vi "Write File.vi"(8 "error in":errorcluster, 10 "Data In":refnum<class "Data.lvclass">, 11 "File Obs in":refnum<class "CRD File Obs.lvclass">) -> (0 "error out":errorcluster, 3 "File Obs out":refnum<class "CRD File Obs.lvclass">)   [LabVIEW 2014, in "CRD File Obs.lvclass"]
uses:
  CRD File Obs.lvclass
  Data/Main/crd_data_enum.ctl
  Data/Main/CRDS Data.lvclass
  Data/Data.lvclass
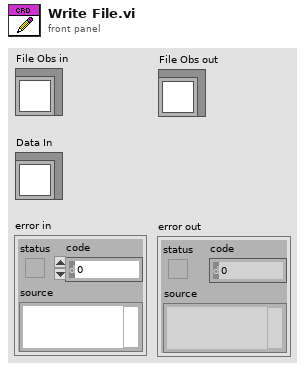
[diagram p1: front panel]
types:
  T1 = typedef "crd_data_enum.ctl" = enum8{"Time", "RHw", "TRH", "P", "Tmean", "RHsense", "TQ", "PQ", "Q", "Q0", "Qcal", "Qset", "extDilFac", "taucorr", "tau0corr", "stdevtau", "ext", "extCorr", "etau", "tau", "tau0", "Purge_Data", "NoData", "reserved", "Ttec", "Ang Exp", "Gamma", "filter", "fOverride", "notes", "max amp", "Tthermistor", "RhdilFac", "Psense", "TRHsense_bank", "RHsense_bank", "MFC_Data", "Thum", "ThumSP", "O3 Flow", "Pinlet Flow", "CLAP Flow", "O3 Add Valve", "O2 Valve", "O3 Cal"}
  T2 = enum16{"big-endian, network order", "native, host order", "little-endian"}
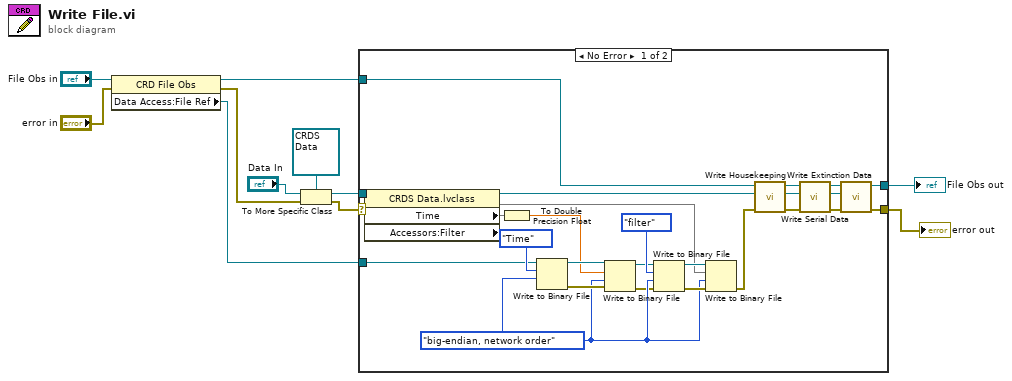
[diagram p0: block diagram]
diagram:
  n1 = property class="CRD File Obs"(reference="File Obs in", error in="error in") -> (reference out=w6:refnum<class "CRD File Obs.lvclass">, error out=w3:errorcluster, "Data Access:File Ref"=w7:refnum<file>)
  n2 = To More Specific Class(target class=refnum<class "CRDS Data.lvclass"> refnum ("CRDS Data in"), reference="Data In", error in=w3) -> (specific class reference=w9:refnum<class "CRDS Data.lvclass">, error out=w2:errorcluster)
  n3 = case shown="No Error" w2 {
    selector: w2 -> [w14 w39]
    tunnel: [w16 w39] -> w4
    tunnel: w9 -> [w30 _]
    tunnel: w7 -> [w13 _]
    tunnel: w6 -> [w24 w38]
    tunnel: [w15 w38] -> w5
    frame No Error {
      w28 = T2."big-endian, network order" ("byte order (0:big-endian, network order)")
      n4 = property class="CRDS Data.lvclass"(reference=w30, error in=w14) -> (reference out=w25:refnum<class "CRDS Data.lvclass">, "Time"=w29, "Accessors:Filter"=w12)  [unwired: 1 out]
      n5 = To Double Precision Float(number=w29) -> (double precision float=w34:dbl)
      n6 = Write to Binary File(file (use dialog)=w13, data=crd_data_enum."Time" ("CRD_Data_Enum"), 9:w28) -> (refnum out=w35:refnum<file>, error out=w36:errorcluster)  [unwired: 3 in, 1 out]
      n7 = Write to Binary File(file (use dialog)=w35, data=w34, error in=w36, 9:w28) -> (refnum out=w27:refnum<file>, error out=w26:errorcluster)  [unwired: 2 in, 1 out]
      n8 = Write to Binary File(file (use dialog)=w27, data=crd_data_enum."filter" ("CRD_Data_Enum"), error in=w26, 9:w28) -> (refnum out=w32:refnum<file>, error out=w31:errorcluster)  [unwired: 2 in, 1 out]
      n9 = Write to Binary File(file (use dialog)=w32, data=w12, error in=w31, 9:w28) -> (error out=w20:errorcluster)  [unwired: 2 in, 2 out]
      n10 = call "Write Housekeeping.vi"("error in"=w20, "CRDS Data in"=w25, "File Obs in"=w24) -> ("error out"=w21:errorcluster, "CRD Data Out"=w23:refnum<class "CRDS Data.lvclass">, "File Obs Out"=w22:refnum<class "CRD File Obs.lvclass">)  [unwired: 6 in]
      n11 = call "Write Serial Data.vi"("error in"=w21, "CRD Data In"=w23, "File Obs in"=w22) -> ("error out"=w17:errorcluster, "CRD Data Out"=w18:refnum<class "CRDS Data.lvclass">, "File Obs Out"=w19:refnum<class "CRD File Obs.lvclass">)  [unwired: 6 in]
      n12 = call "Write Extinction Data.vi"("error in"=w17, "CRDS Data in"=w18, "CRD File Obs in"=w19) -> ("error out"=w16:errorcluster, "CRD File Obs out"=w15:refnum<class "CRD File Obs.lvclass">)  [unwired: 7 in]
    }
    frame Error {
    }
  }
  "error out" <- w4
  "File Obs out" <- w5
